vi "VCS Get Device Error Code.vi"(8 "error in (no error)":errorcluster, 10 "Error Number":u8=1 min=1 max=9, 11 "axis In":cluster{"keyHandle":u32, "nodeId":u16}={"keyHandle"=0, "nodeId"=1}) -> (0 "error out":errorcluster, 1 "Error Code":u32, 3 "axis Out":cluster{"keyHandle":u32, "nodeId":u16}={"keyHandle"=0, "nodeId"=1})   [LabVIEW 2019, in "maxonEPOS.lvlib"]
doc: "<B>VCS Get Device Error Code</B> returns the error code of the given error history index."
uses:
  Examples/maxonEPOS.lvlib
  Resources/EposCmd.dll
  Resources/EposCmd64.dll
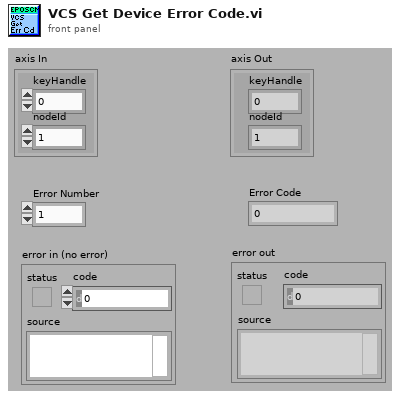
[diagram p1: front panel]
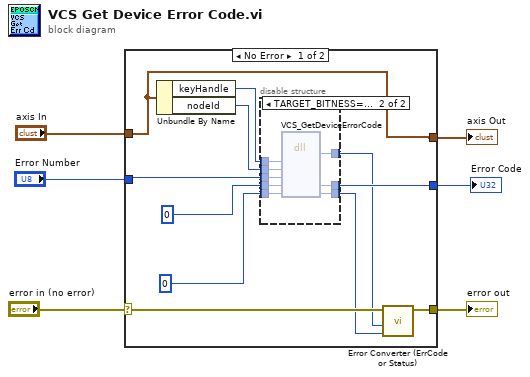
[diagram p0: block diagram]
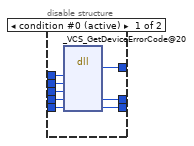
[diagram p2: hidden frame]
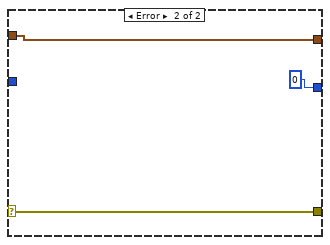
[diagram p3: hidden frame]
diagram:
  n1 = case shown="No Error" "error in (no error)" {
    selector: "error in (no error)" -> [w17 w36]
    tunnel: [w16 w36] -> w5
    tunnel: "axis In" -> [w13 w35]
    tunnel: [w13 w35] -> w3
    tunnel: "Error Number" -> [w12 _]
    tunnel: [w8 u8 0 ("pNbDeviceError")] -> w1
    frame No Error {
      n2 = Unbundle By Name(w13) -> ("keyHandle"=w15:u32, "nodeId"=w14:u16)
      n3 = disable-structure shown="TARGET_BITNESS==64" {
        disable-tunnel: w15 -> [w25 w33]
        disable-tunnel: w14 -> [w24 w32]
        disable-tunnel: w12 -> [w23 w31]
        disable-tunnel: [w22 w28] -> w11
        disable-tunnel: u32 0 ("pErrorCode") -> [w21 w29]
        disable-tunnel: u32 0 ("pErrorCode") -> [w20 w30]
        disable-tunnel: [w19 w27] -> w8
        disable-tunnel: [w18 w26] -> w7
        frame condition #0 (active) {
          n4 = dll-call lib="C:/workspace/project/scancon/sw/SSI_Tool/InstrumentsInterfaces/Motordriver/maxon EPOS/Resources/EposCmd.dll" fn="_VCS_GetDeviceErrorCode@20" ("EposCmd.dll:_VCS_GetVersion@28")("KeyHandle"=w25, "NodeId"=w24, "SubIndex"=w23, "pDeviceErrorCode"=w20, "pErrorCode"=w21) -> ("Rückgabetyp"=w18:i32, "pDeviceErrorCode"=w19:u32, "pErrorCode"=w22:u32)  [unwired: 6 in, 2 out]
        }
        frame condition #1 {
          n5 = dll-call lib="C:/Sources/LabView/maxon EPOS/Resources/EposCmd64.dll" fn="VCS_GetDeviceErrorCode" ("EposCmd.dll:_VCS_GetVersion@28")("KeyHandle"=w33, "NodeId"=w32, "SubIndex"=w31, "pDeviceErrorCode"=w30, "pErrorCode"=w29) -> ("Rückgabetyp"=w26:i32, "pDeviceErrorCode"=w27:u32, "pErrorCode"=w28:u32)  [unwired: 6 in, 2 out]
        }
      }
      n6 = call "Error Converter (ErrCode or Status).vi"("error code"=w11, "return type"=w7, "error in (no error)"=w17) -> ("error out"=w16:errorcluster)  [unwired: 7 in]
    }
    frame Error {
    }
  }
  "error out" <- w5
  "axis Out" <- w3
  "Error Code" <- w1
